vi "test_TrajectoryTS090820Circular2D.vi"() -> ()   [LabVIEW 2010, in "TrajectoryTS090820Circular2D.lvclass"]
uses:
  TrajectoryTS090820Circular2D.lvclass
  TrajectoryTS090820Circular2D.lvclass/TrajectoryTS090820Circular2D.ctl
panel:
  in  "generate double circle":bool
  in  "rotation angle":dbl
  in  "y center":dbl
  in  "x center":dbl
  in  "total number of pixels per cycle":i32=1000
  in  "Phase shift":dbl
  in  "y frequency":dbl=1.0
  in  "x frequency":dbl=1.0
  in  "y amplitude":dbl[unit]=4.9999999999999996e-05
  in  "x amplitude":dbl[unit]=4.9999999999999996e-05
  in  "generate button":bool
  in  "stop button":bool
  out "coordinates":dbl[unit][][](graph)
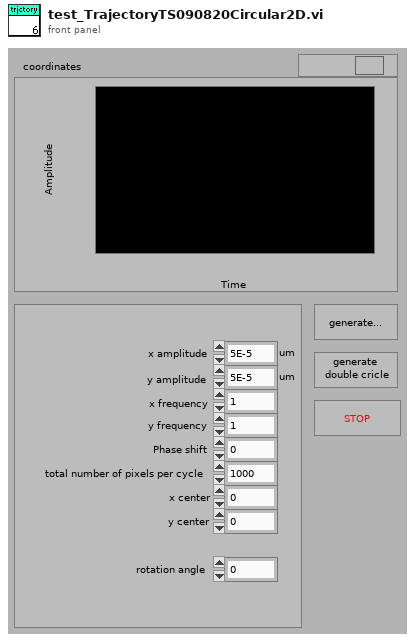
[diagram p1: front panel]
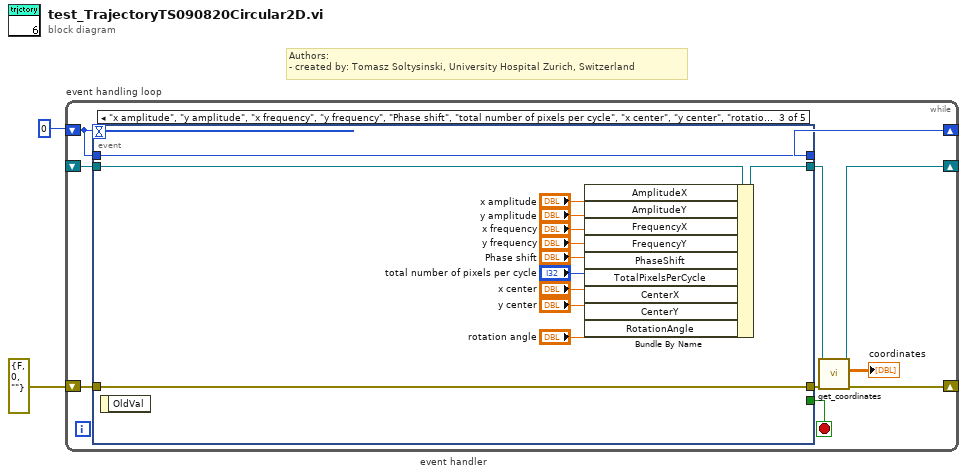
[diagram p0: block diagram]
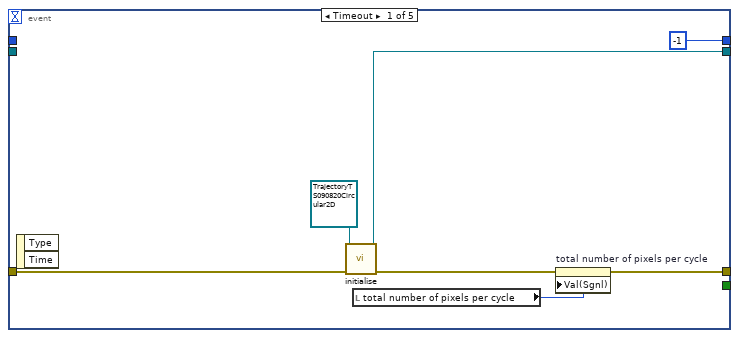
[diagram p2: hidden frame]
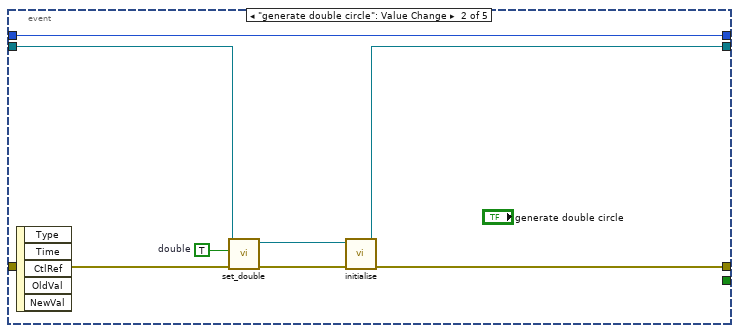
[diagram p3: hidden frame]
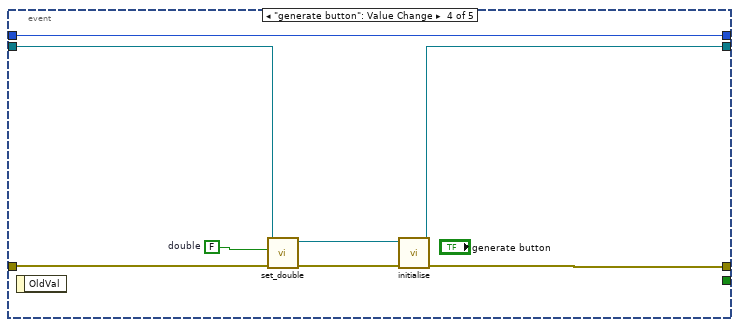
[diagram p4: hidden frame]
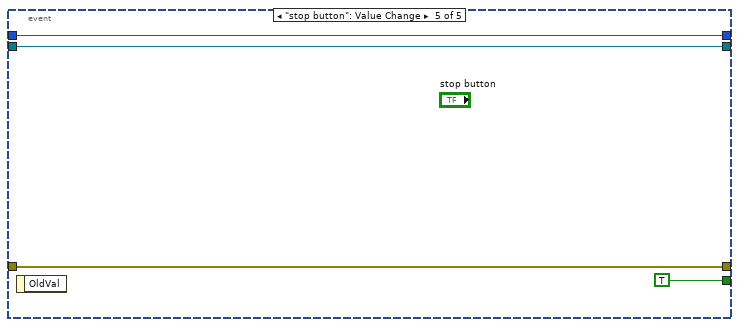
[diagram p5: hidden frame]
diagram:
  # "Authors: \n- created by: Tomasz Soltysinski, University Hospital Zurich, Switzerland"
  n1 = while "event handling loop" {
    shift-right: [w10] -> _
    shift-left: 0 -> [w11]
    shift-right: [w6] -> _
    shift-left: errorcluster {"status"=FALSE, "code"=0, "source"=""} ("error in (no error)") -> [w12]
    shift-right: [w4] -> _
    shift-left: _ -> [w9]
    stop <- w8 stop-if-true
    n2 = event "event handler" shown="[2] \"x amplitude\", \"y amplitude\", \"x frequency\", \"y frequency\", \"Phase shift\", \"total number of pixels per cycle\", \"x center\", \"y center\", \"rotation angle\": Value Change" {
      selector: _ -> [_ _ _ _ _]
      dyn-events: _ -> [_ _ _ _ _]
      timeout: w11 -> [_ _ _ _ _]
      tunnel: w12 -> [w19 w22 w40 w42 w52]
      tunnel: w11 -> [_ w27 w39 w48 w51]
      tunnel: [w13 w25 w40 w46 w52] -> w5
      tunnel: [-1 w27 w39 w48 w51] -> w10
      tunnel: [w16 w26 w37 w47 w50] -> w3
      tunnel: w9 -> [_ w24 w38 w44 w50]
      tunnel: [_ _ _ _ TRUE] -> w8
      event Timeout {
        n3 = event-data() -> ()  [unwired: 1 in, 2 out]
        n4 = call-dynamic "initialise.vi"("error in (no error)"=w19, "TrajectoryTS090820Circular2D in"=refnum<class "TrajectoryTS090820Circular2D.lvclass"> refnum ("TrajectoryTS090820Circular2D.lvclass")) -> ("error out"=w14:errorcluster, "TrajectoryTS090820Circular2D out"=w16:refnum<class "TrajectoryTS090820Circular2D.lvclass">)  [unwired: 8 in]
        n5 = local read "total number of pixels per cycle"() -> (w15:i32)
        n6 = property on="total number of pixels per cycle" class="DigNum (strict)"(error in=w14, "Val(Sgnl)"=w15) -> (error out=w13:errorcluster)  [unwired: 1 in, 1 out]
      }
      event "generate double circle": Value Change {
        w20 = TRUE  # double
        n7 = event-data() -> ()  [unwired: 1 in, 5 out]
        n8 = call-dynamic "set_double.vi"("error in (no error)"=w22, "double"=w20, "TrajectoryTS090820Circular2D in"=w24) -> ("error out"=w21:errorcluster, "TrajectoryTS090820Circular2D out"=w23:refnum<class "TrajectoryTS090820Circular2D.lvclass">)  [unwired: 7 in]
        n9 = call-dynamic "initialise.vi"("error in (no error)"=w21, "TrajectoryTS090820Circular2D in"=w23) -> ("error out"=w25:errorcluster, "TrajectoryTS090820Circular2D out"=w26:refnum<class "TrajectoryTS090820Circular2D.lvclass">)  [unwired: 8 in]
      }
      event "x amplitude", "y amplitude", "x frequency", "y frequency", "Phase shift", "total number of pixels per cycle", "x center", "y center", "rotation angle": Value Change {
        n10 = event-data() -> ()  [unwired: 1 in, 1 out]
        n11 = Bundle By Name(cluster=w38, "AmplitudeX"="x amplitude", "AmplitudeY"="y amplitude", "FrequencyX"="x frequency", "FrequencyY"="y frequency", "PhaseShift"="Phase shift", "TotalPixelsPerCycle"="total number of pixels per cycle", "CenterX"="x center", "CenterY"="y center", "RotationAngle"="rotation angle") -> (w37:refnum<class "TrajectoryTS090820Circular2D.lvclass">)
      }
      event "generate button": Value Change {
        w45 = FALSE  # double
        n12 = event-data() -> ()  [unwired: 1 in, 1 out]
        n13 = call-dynamic "set_double.vi"("error in (no error)"=w42, "double"=w45, "TrajectoryTS090820Circular2D in"=w44) -> ("error out"=w41:errorcluster, "TrajectoryTS090820Circular2D out"=w43:refnum<class "TrajectoryTS090820Circular2D.lvclass">)  [unwired: 7 in]
        n14 = call-dynamic "initialise.vi"("error in (no error)"=w41, "TrajectoryTS090820Circular2D in"=w43) -> ("error out"=w46:errorcluster, "TrajectoryTS090820Circular2D out"=w47:refnum<class "TrajectoryTS090820Circular2D.lvclass">)  [unwired: 8 in]
      }
      event "stop button": Value Change {
        n15 = event-data() -> ()  [unwired: 1 in, 1 out]
      }
    }
    n16 = call-dynamic "get_coordinates.vi"("error in (no error)"=w5, "GenericTrajectory in"=w3) -> ("error out"=w6:errorcluster, "coordinates"=→"coordinates":dbl[unit][][], "GenericTrajectory out"=w4:refnum<class "TrajectoryTS090820Circular2D.lvclass">)  [unwired: 7 in]
  }
